vi "stopWMPStream.vi"(8 "error in (no error)":errorcluster, 10 "stop":bool, 11 "SoundAO in":refnum<class "SoundAO.lvclass">) -> (0 "error out":errorcluster, 2 "Stopped":bool, 3 "SoundAO out":refnum<class "SoundAO.lvclass">)   [LabVIEW 2009, in "Hardware.lvlib" / "Channels.lvlib" / "SoundAO.lvclass"]
uses:
  SoundAO.lvclass
  SoundAO.lvclass/SoundAO.ctl
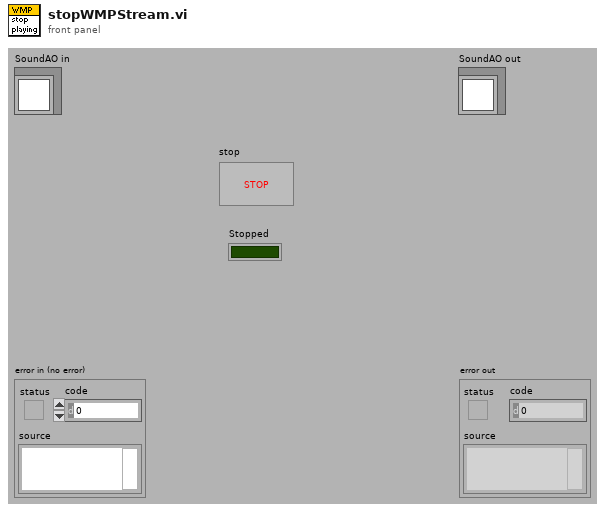
[diagram p1: front panel]
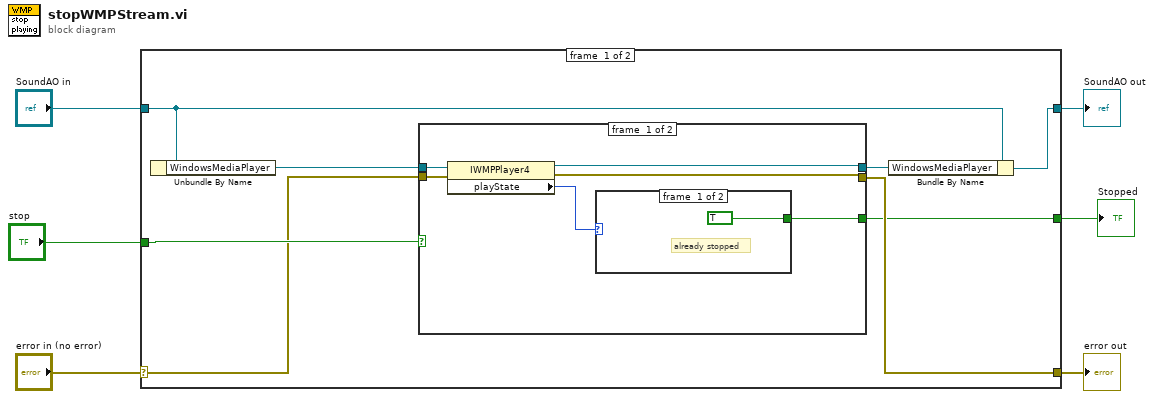
[diagram p0: block diagram]
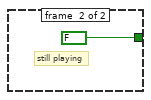
[diagram p2: hidden frame]
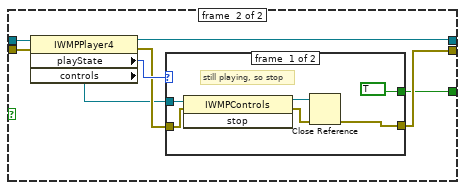
[diagram p3: hidden frame]
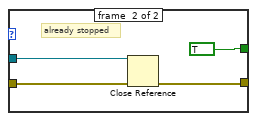
[diagram p4: hidden frame]
diagram:
  n1 = case shown="No Error" "error in (no error)" {
    selector: "error in (no error)" -> [w8 w42]
    tunnel: [w14 w42] -> w5
    tunnel: [w12 w41] -> w3
    tunnel: "SoundAO in" -> [w13 w41]
    tunnel: "stop" -> [w11 _]
    tunnel: [w7 _] -> w1
    frame #0 {
      n2 = Unbundle By Name(w13) -> ("WindowsMediaPlayer"=w9:refnum<k7>)
      n3 = case shown="True" w11 {
        tunnel: [w17 w30] -> w14
        tunnel: w9 -> [w20 w29]
        tunnel: w8 -> [w19 w28]
        tunnel: [w18 w25] -> w10
        tunnel: [w15 w23] -> w7
        frame #0 {
          n4 = property class="IWMPPlayer4"(reference=w20, error in=w19) -> (reference out=w18:refnum<k7>, error out=w17:errorcluster, "playState"=w16:i32)
          n5 = case shown="1" w16 {
            tunnel: [TRUE FALSE] -> w15
            frame #0 {
              # "already stopped"
            }
            frame #1 {
              # "still playing"
            }
          }
        }
        frame #1 {
          n6 = property class="IWMPPlayer4"(reference=w29, error in=w28) -> (reference out=w25:refnum<k7>, error out=w26:errorcluster, "playState"=w27:i32, "controls"=w24:refnum<k7>)
          n7 = case shown="Default" w27 {
            tunnel: [w34 w39] -> w30
            tunnel: w24 -> [w33 w40]
            tunnel: w26 -> [w32 w38]
            tunnel: [TRUE TRUE] -> w23
            frame #0 {
              # "still playing, so stop"
              n8 = invoke class="IWMPControls" method="stop"(reference=w33, error in=w32) -> (reference out=w36:refnum<k7>, error out=w35:errorcluster)  [unwired: 1 in, 1 out]
              n9 = Close Reference(reference=w36, error in (no error)=w35) -> (error out=w34:errorcluster)
            }
            frame #1 {
              # "already stopped"
              n10 = Close Reference(reference=w40, error in (no error)=w38) -> (error out=w39:errorcluster)
            }
          }
        }
      }
      n11 = Bundle By Name(cluster=w13, "WindowsMediaPlayer"=w10) -> (w12:refnum<class "SoundAO.lvclass">)
    }
    frame #1 {
    }
  }
  "error out" <- w5
  "SoundAO out" <- w3
  "Stopped" <- w1
